vi "Ticks To Degrees.vi"(11 "Position (ticks)":dbl) -> (3 "Position (degrees)":dbl)   [LabVIEW 2020]
doc: "unit conversion: ticks --> degrees (cancoder units)"
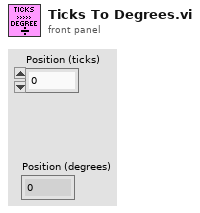
[diagram p1: front panel]
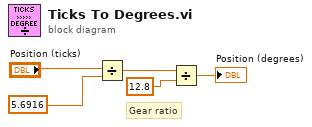
[diagram p0: block diagram]
diagram:
  # "Gear ratio"
  n1 = Divide(x="Position (ticks)", y=5.6916 ("Scale Factor")) -> (x/y=w3:dbl)
  n2 = Divide(x=w3, y=12.8) -> (x/y=→"Position (degrees)":dbl)
